vi "HEWH Check Voltage.vi"(8 "error in (no error)":errorcluster, 11 "UEF Calculated Values Input":T1 {"Data Indexes"."15 sec after Draw Index" format="%#.2f"; "Data Indexes"."15 sec after Draw Timestamp" format="%#.2f"; "Data Indexes"."Test Start Timestamp" format="%.2f"; "Data Indexes"."Test End Timestamp" format="%.2f"; "Data Indexes"."T0 Timestamp" format="%.2f"; "Data Indexes"."Tsf Timestamp" format="%.2f"; "Data Indexes"."Tsu0 Timestamp" format="%.2f"; "Data Indexes"."Tmax1 Timestamp" format="%.2f"; "Data Indexes"."Draw Index Timestamp" format="%#.2f"; "Data Indexes"."Non-Draw Timestamp" format="%#.2f"; "Data Indexes"."Heating Timestamp" format="%#.2f"; "Data Indexes"."Start Energy (BTU-Gas)" format="%.6f"; "Data Indexes"."Start Watt Hours" format="%.6f"; "Static Data"."V - Volume of Wh (True)" format="%.5f"; "Static Data"."T-Ambinet Nominal (°F)" format="%.5f"; "Static Data"."T-Inlet Setpoint (°F)" format="%.5f"; "Static Data"."T-Wh Setpoint (°F)" format="%.5f"; "Sampled Data"."Qe (Wh)" format="%.5f"; "Sampled Data"."Tau stby2 (hr)" format="%.5f"; "Sampled Data"."Tastby2 (°F)" format="%.5f"; "Sampled Data"."Qf (BTU)" format="%.5f"; "Sampled Data"."Qe (BTU)" format="%.5f"; "Sampled Data"."Tmax1 (°F)" format="%.5f"; "Sampled Data"."T0 (°F)" format="%.5f"; "Sampled Data"."Qr (BTU)" format="%.5f"; "Sampled Data"."T 24(°F)" format="%.5f"; "Sampled Data"."T astby(°F)" format="%.5f"; "Sampled Data"."T tstby(°F)" format="%.5f"; "Sampled Data"."T su0(°F)" format="%.5f"; "Sampled Data"."T suf(°F)" format="%.5f"; "Sampled Data"."Tau stby_1 (hr)" format="%.5f"; "Sampled Data"."Qsuf (BTU)" format="%.5f"; "Sampled Data"."Qsu0 (BTU)" format="%.5f"; "Calculated Values"."Draw Bonus Volume (gal)" format="%.6f"; "Calculated Values"."Adjustment Factor" format="%.6f"; "Calculated Values"."T*avg_del(n-1)" format="%.6f"; "Calculated Values"."T*min(n-1)" format="%.6f"; "Calculated Values"."T*avg_del(n)" format="%.6f"; "Calculated Values"."Vn" format="%.6f"; "Calculated Values"."Qdm (BTU)" format="%.6f"; "Calculated Values"."QHWD (BTU)" format="%.6f"; "Calculated Values"."QHW (BTU)" format="%.6f"; "Calculated Values"."UEF" format="%.6f"; "Calculated Values"."QHW67 (BTU)" format="%.6f"; "Calculated Values"."Qda (BTU)" format="%.6f"; "Calculated Values"."Qd (BTU)" format="%.6f"; "Calculated Values"."Q (BTU)" format="%.6f"; "Calculated Values"."UA (BTU/(hr*F))" format="%.6f"; "Calculated Values"."Qhr (BTU/hr)" format="%.6f"; "Calculated Values"."Qstby (BTU)" format="%.6f"; "Calculated Values"."nu_r" format="%.6f"; "Calculated Values"."CpUEF (BTU/(lb*F))" format="%.6f"; "Calculated Values"."rho_nu (lb/gal)" format="%.6f"; "Calculated Values"."V1- Vol (Gal)" format="%.6f"; "Calculated Values"."M cluster mass removed (lb)" format="%.6f"; "Calculated Values"."Cp theoretical (BTU/(lbm °F))" format="%.6f"; "Calculated Values"."Tin1 - Mean Inlet 1st Cluster (°F)" format="%.6f"; "Calculated Values"."Tdel1-Mean Outlet 1st Cluster(°F)" format="%.6f"; "Calculated Values"."Cp 24 (BTU/(lb*F))" format="%.6f"; "Calculated Values"."Cp standby (BTU/(lb*F))" format="%.6f"; "Calculated Values"."Cp2 (BTU/(lb*F))" format="%.6f"; "Calculated Values"."Cp1 (BTU/(lb*F))" format="%.6f"; "Calculated Values"."rho 24 (lb/gal)" format="%.6f"; "Calculated Values"."rho standby (lb/gal)" format="%.6f"; "Calculated Values"."rho 2 (lb/gal)" format="%.6f"; "Calculated Values"."Density of cold water All (lbm/gal)" format="%#.3g"; "Calculated Values"."CpHW (BTU/(lbm °F))" format="%#.3g"; "Calculated Values"."Density of hot water All (lbm/gal)" format="%#.3g"; "Calculated Values"."Mass of water All (lbm)" format="%#.3f"}) -> (0 "error out":errorcluster, 3 "UEF Calculated Values Output":T1 {"Data Indexes"."15 sec after Draw Index" format="%#.2f"; "Data Indexes"."15 sec after Draw Timestamp" format="%#.2f"; "Data Indexes"."Test Start Timestamp" format="%.2f"; "Data Indexes"."Test End Timestamp" format="%.2f"; "Data Indexes"."T0 Timestamp" format="%.2f"; "Data Indexes"."Tsf Timestamp" format="%.2f"; "Data Indexes"."Tsu0 Timestamp" format="%.2f"; "Data Indexes"."Tmax1 Timestamp" format="%.2f"; "Data Indexes"."Draw Index Timestamp" format="%#.2f"; "Data Indexes"."Non-Draw Timestamp" format="%#.2f"; "Data Indexes"."Heating Timestamp" format="%#.2f"; "Data Indexes"."Start Energy (BTU-Gas)" format="%.6f"; "Data Indexes"."Start Watt Hours" format="%.6f"; "Static Data"."V - Volume of Wh (True)" format="%.5f"; "Static Data"."T-Ambinet Nominal (°F)" format="%.5f"; "Static Data"."T-Inlet Setpoint (°F)" format="%.5f"; "Static Data"."T-Wh Setpoint (°F)" format="%.5f"; "Sampled Data"."Qe (Wh)" format="%.5f"; "Sampled Data"."Tau stby2 (hr)" format="%.5f"; "Sampled Data"."Tastby2 (°F)" format="%.5f"; "Sampled Data"."Qf (BTU)" format="%.5f"; "Sampled Data"."Qe (BTU)" format="%.5f"; "Sampled Data"."Tmax1 (°F)" format="%.5f"; "Sampled Data"."T0 (°F)" format="%.5f"; "Sampled Data"."Qr (BTU)" format="%.5f"; "Sampled Data"."T 24(°F)" format="%.5f"; "Sampled Data"."T astby(°F)" format="%.5f"; "Sampled Data"."T tstby(°F)" format="%.5f"; "Sampled Data"."T su0(°F)" format="%.5f"; "Sampled Data"."T suf(°F)" format="%.5f"; "Sampled Data"."Tau stby_1 (hr)" format="%.5f"; "Sampled Data"."Qsuf (BTU)" format="%.5f"; "Sampled Data"."Qsu0 (BTU)" format="%.5f"; "Calculated Values"."Draw Bonus Volume (gal)" format="%.6f"; "Calculated Values"."Adjustment Factor" format="%.6f"; "Calculated Values"."T*avg_del(n-1)" format="%.6f"; "Calculated Values"."T*min(n-1)" format="%.6f"; "Calculated Values"."T*avg_del(n)" format="%.6f"; "Calculated Values"."Vn" format="%.6f"; "Calculated Values"."Qdm (BTU)" format="%.6f"; "Calculated Values"."QHWD (BTU)" format="%.6f"; "Calculated Values"."QHW (BTU)" format="%.6f"; "Calculated Values"."UEF" format="%.6f"; "Calculated Values"."QHW67 (BTU)" format="%.6f"; "Calculated Values"."Qda (BTU)" format="%.6f"; "Calculated Values"."Qd (BTU)" format="%.6f"; "Calculated Values"."Q (BTU)" format="%.6f"; "Calculated Values"."UA (BTU/(hr*F))" format="%.6f"; "Calculated Values"."Qhr (BTU/hr)" format="%.6f"; "Calculated Values"."Qstby (BTU)" format="%.6f"; "Calculated Values"."nu_r" format="%.6f"; "Calculated Values"."CpUEF (BTU/(lb*F))" format="%.6f"; "Calculated Values"."rho_nu (lb/gal)" format="%.6f"; "Calculated Values"."V1- Vol (Gal)" format="%.6f"; "Calculated Values"."M cluster mass removed (lb)" format="%.6f"; "Calculated Values"."Cp theoretical (BTU/(lbm °F))" format="%.6f"; "Calculated Values"."Tin1 - Mean Inlet 1st Cluster (°F)" format="%.6f"; "Calculated Values"."Tdel1-Mean Outlet 1st Cluster(°F)" format="%.6f"; "Calculated Values"."Cp 24 (BTU/(lb*F))" format="%.6f"; "Calculated Values"."Cp standby (BTU/(lb*F))" format="%.6f"; "Calculated Values"."Cp2 (BTU/(lb*F))" format="%.6f"; "Calculated Values"."Cp1 (BTU/(lb*F))" format="%.6f"; "Calculated Values"."rho 24 (lb/gal)" format="%.6f"; "Calculated Values"."rho standby (lb/gal)" format="%.6f"; "Calculated Values"."rho 2 (lb/gal)" format="%.6f"; "Calculated Values"."Density of cold water All (lbm/gal)" format="%#.3g"; "Calculated Values"."CpHW (BTU/(lbm °F))" format="%#.3g"; "Calculated Values"."Density of hot water All (lbm/gal)" format="%#.3g"; "Calculated Values"."Mass of water All (lbm)" format="%#.3f"})   [LabVIEW 2023]
uses:
  Type Definitions/UEF Constants.ctl
  Type Definitions/HEWH Draw Stats.ctl
  Type Definitions/HEWH FHR Draw Type.ctl
  Type Definitions/FHR Bins.ctl
  Type Definitions/HEWH Meter Type.ctl
  Type Definitions/HEWH Seconds to Remove.ctl
  Type Definitions/HEWH Remove From Location.ctl
panel:
  # "FHR"
  # "FHR"
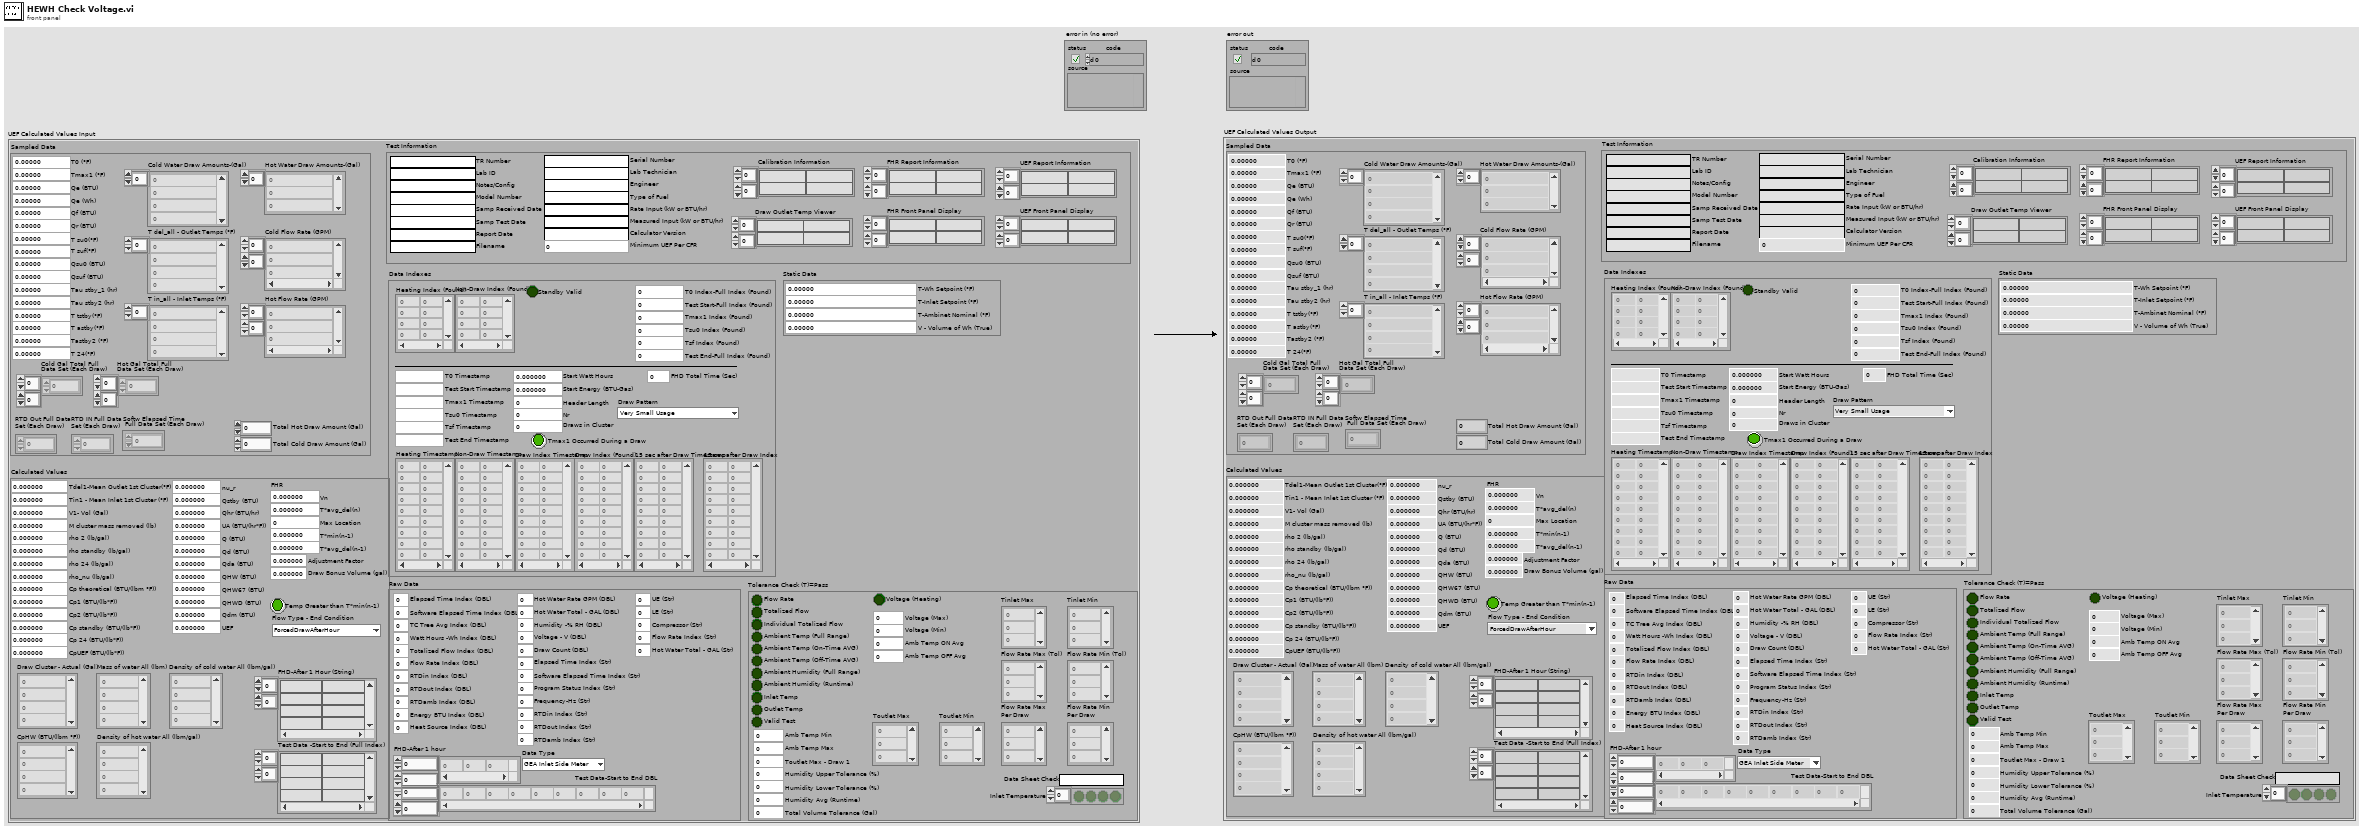
[diagram p1: front panel]
types:
  T1 = typedef "UEF Constants.ctl" = cluster{"Calculated Values":T2, "Sampled Data":cluster{"Cold Water Draw Amounts-(Gal)":dbl[], "T del_all - Outlet Temps (°F)":dbl[], "T in_all - Inlet Temps (°F)":dbl[], "Qsu0 (BTU)":dbl, "Qsuf (BTU)":dbl, "Tau stby_1 (hr)":dbl, "T suf(°F)":dbl, "T su0(°F)":dbl, "T tstby(°F)":dbl, "T astby(°F)":dbl, "T 24(°F)":dbl, "Qr (BTU)":dbl, "T0 (°F)":dbl, "Tmax1 (°F)":dbl, "Qe (BTU)":dbl, "Qf (BTU)":dbl, "Tastby2 (°F)":dbl, "RTD Out Full Data\nSet (Each Draw)":dbl[][], "RTD IN Full Data\nSet (Each Draw)":dbl[][], "Tau stby2 (hr)":dbl, "Hot Water Draw Amounts-(Gal)":dbl[], "Cold Flow Rate (GPM)":dbl[][], "Hot Flow Rate (GPM)":dbl[][], "Softw Elapsed Time\n Full Data Set (Each Draw)":dbl[][], "Cold Gal Total Full\nData Set (Each Draw)":dbl[][], "Total Hot Draw Amount (Gal) ":dbl, "Total Cold Draw Amount (Gal)":dbl, "Qe (Wh)":dbl, "Hot Gal Total Full\nData Set (Each Draw)":dbl[][]}, "Static Data":cluster{"T-Wh Setpoint (°F)":dbl, "T-Inlet Setpoint (°F)":dbl, "T-Ambinet Nominal (°F)":dbl, "V - Volume of Wh (True)":dbl}, "Data Indexes":cluster{"Test Start-Full Index (Found)":i32, "Header Length":i32, "Draw Index (Found)":i32[][], "Nr":i32, "Start Watt Hours":dbl, "Tsu0 Index (Found)":i32, "Tsf Index (Found)":i32, "Start Energy (BTU-Gas)":dbl, "Draws in Cluster":i32, "T0 Index-Full Index (Found)":i32, "Non-Draw Index (Found)":i32[][], "Tmax1 Index (Found)":i32, "Test End-Full Index (Found)":i32, "Heating Index (Found)":i32[][], "Heating Timestamp":dbl[][], "Non-Draw Timestamp":dbl[][], "Draw Index Timestamp":dbl[][], "Tmax1 Timestamp":dbl, "Tsu0 Timestamp":dbl, "Tsf Timestamp":dbl, "T0 Timestamp":dbl, "Test End Timestamp":dbl, "Test Start Timestamp":dbl, "15 sec after Draw Timestamp":dbl[][], "15 sec after Draw Index":dbl[][], "Tmax1 Occurred During a Draw":bool, "FHD Total Time (Sec)":dbl, "Draw Pattern":T4, "Standby Valid":bool}, "Raw Data":cluster{"Elapsed Time Index (DBL)":i32, "Software Elapsed Time Index (DBL)":i32, "TC Tree Avg Index (DBL)":i32, "Watt Hours -Wh Index (DBL)":i32, "Energy BTU Index (DBL)":i32, "Totalized Flow Index (DBL)":i32, "Flow Rate Index (DBL)":i32, "Program Status Index (Str)":i32, "RTDin Index (DBL)":i32, "RTDout Index (DBL)":i32, "RTDamb Index (DBL)":i32, "Test Data-Start to End DBL":dbl[][], "Data Type":T5, "Heat Source Index (DBL)":i32, "Hot Water Rate GPM (DBL)":i32, "Hot Water Total - GAL (DBL)":i32, "FHD-After 1 hour":dbl[][], "Humidity -% RH (DBL)":i32, "Voltage - V (DBL)":i32, "Draw Count (DBL)":i32, "Elapsed Time Index (Str)":i32, "Software Elapsed Time Index (Str)":i32, "Frequency-Hz (Str)":i32, "RTDin Index (Str)":i32, "RTDout Index (Str)":i32, "RTDamb Index (Str)":i32, "UE (Str)":i32, "LE (Str)":i32, "Compressor (Str)":i32, "Flow Rate Index (Str)":i32, "Hot Water Total - GAL (Str)":i32}, "Tolerance Check (T)=Pass":cluster{"Flow Rate":bool, "Totalized Flow":bool, "Ambient Temp (Full Range)":bool, "Ambient Humidity (Full Range)":bool, "Inlet Temp":bool, "Outlet Temp":bool, "Valid Test":bool, "Individual Totalized Flow":bool, "Data Sheet Check":string, "Inlet Temperature":bool[], "Tinlet Max":dbl[], "Tinlet Min":dbl[], "Flow Rate Max (Tol)":dbl[], "Flow Rate Min (Tol)":dbl[], "Amb Temp Max":dbl, "Amb Temp Min":dbl, "Toutlet Max - Draw 1":dbl, "Humidity Upper Tolerance (%)":dbl, "Total Volume Tolerance (Gal)":dbl, "Humidity Lower Tolerance (%)":dbl, "Flow Rate Max\nPer Draw":dbl[], "Flow Rate Min\nPer Draw":dbl[], "Ambient Humidity (Runtime)":bool, "Humidity Avg (Runtime)":dbl, "Ambient Temp (On-Time AVG)":bool, "Ambient Temp (Off-Time AVG)":bool, "Amb Temp OFF Avg":dbl, "Amb Temp ON Avg":dbl, "Voltage (Heating)":bool, "Voltage (Min)":dbl, "Voltage (Max)":dbl, "Toutlet Max":dbl[], "Toutlet Min":dbl[]}, "Test Information":cluster{"TR Number":string, "Lab ID":string, "Notes/Config":string, "Model Number":string, "Serial Number":string, "Lab Technician":string, "Engineer":string, "Type of Fuel":string, "Samp Received Date":string, "Samp Test Date":string, "Report Date":string, "Rate Input (kW or BTU/hr)":string, "Measured Input (kW or BTU/hr)":string, "Filename":string, "Calibration Information":string[][], "Calculator Version":string, "Minimum UEF Per CFR":dbl, "UEF Report Information":string[][], "FHR Report Information":string[][], "FHR Front Panel Display":string[][], "UEF Front Panel Display":string[][], "Draw Outlet Temp Viewer":string[][]}}
  T2 = typedef "HEWH Draw Stats.ctl" = cluster{"Draw Cluster - Actual (Gal)":dbl[], "Mass of water All (lbm)":dbl[], "Density of hot water All (lbm/gal)":dbl[], "CpHW (BTU/(lbm °F))":dbl[], "rho 2 (lb/gal)":dbl, "rho standby (lb/gal)":dbl, "rho 24 (lb/gal)":dbl, "Cp1 (BTU/(lb*F))":dbl, "Cp2 (BTU/(lb*F))":dbl, "Cp standby (BTU/(lb*F))":dbl, "Cp 24 (BTU/(lb*F))":dbl, "nu_r":dbl, "Qstby (BTU)":dbl, "Qhr (BTU/hr)":dbl, "UA (BTU/(hr*F))":dbl, "Q (BTU)":dbl, "Qd (BTU)":dbl, "Qda (BTU)":dbl, "QHW67 (BTU)":dbl, "UEF":dbl, "Tdel1-Mean Outlet 1st Cluster(°F)":dbl, "Tin1 - Mean Inlet 1st Cluster (°F)":dbl, "Cp theoretical (BTU/(lbm °F))":dbl, "M cluster mass removed (lb)":dbl, "V1- Vol (Gal)":dbl, "Test Data -Start to End (Full Index)":string[][], "rho_nu (lb/gal)":dbl, "Density of cold water All (lbm/gal)":dbl[], "CpUEF (BTU/(lb*F))":dbl, "QHW (BTU)":dbl, "QHWD (BTU)":dbl, "Qdm (BTU)":dbl, "FHD-After 1 Hour (String)":string[][], "Vn":dbl, "T*avg_del(n)":dbl, "Max Location":i32, "T*min(n-1)":dbl, "T*avg_del(n-1)":dbl, "Temp Greater than T*min(n-1)":bool, "Adjustment Factor":dbl, "Draw Bonus Volume (gal)":dbl, "Flow Type - End Condition":T3}
  T3 = typedef "HEWH FHR Draw Type.ctl" = enum16{"ForcedDrawAfterHour", "HeatingCutoffBeforeHour"}
  T4 = typedef "FHR Bins.ctl" = enum16{"Very Small Usage", "Low Usage", "Medium Usage", "High Usage", "Undefined"}
  T5 = typedef "HEWH Meter Type.ctl" = enum16{"GEA Inlet Side Meter", "GEA Outlet Side Meter", "CSA Inlet Side Meter"}
  T6 = typedef "HEWH Remove From Location.ctl" = enum16{"Remove from  Beginning", "Remove from End"}
  T7 = typedef "HEWH Seconds to Remove.ctl" = enum16{"5 Seconds", "15 Seconds"}
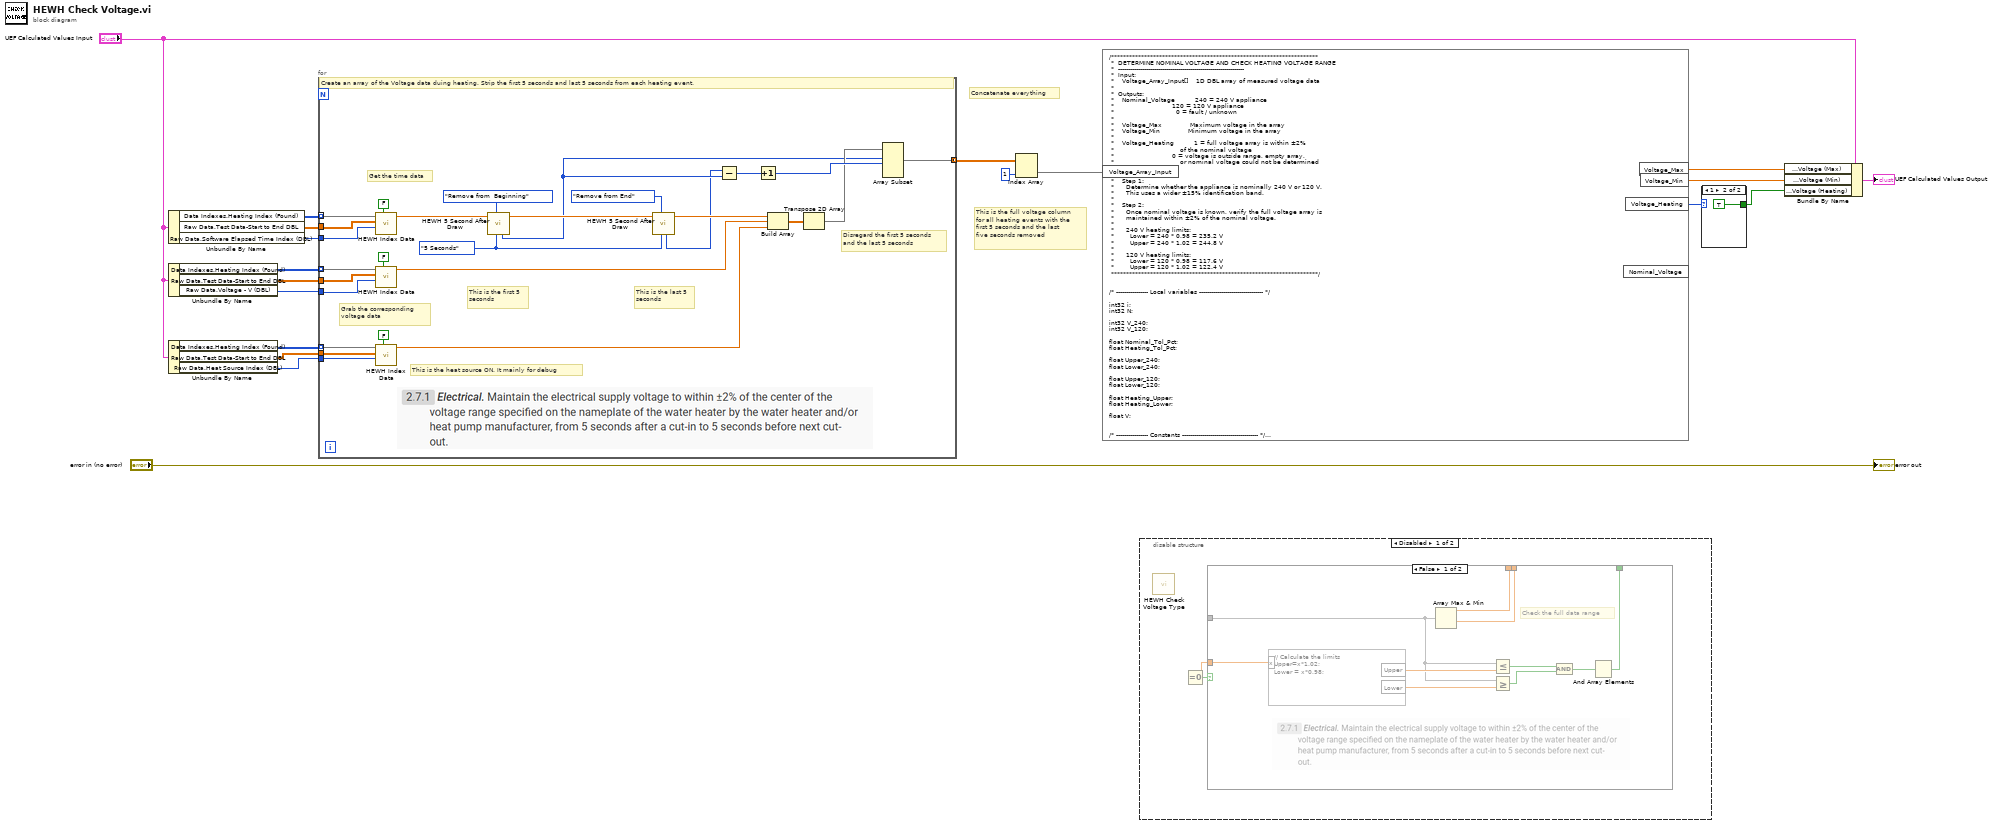
[diagram p0: block diagram]
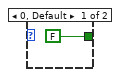
[diagram p2: hidden frame]
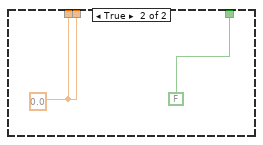
[diagram p3: hidden frame]
diagram:
  # "This is the full voltage column\nfor all heating events with the\nfirst 5 seconds and the last\nfive seconds removed"
  # "Concatenate everything"
  n1 = Unbundle By Name("UEF Calculated Values Input") -> ("Data Indexes.Heating Index (Found)"=w16:i32[][], "Raw Data.Test Data-Start to End DBL"=w15:dbl[][], "Raw Data.Software Elapsed Time Index (DBL)"=w14:i32)
  n2 = Unbundle By Name("UEF Calculated Values Input") -> ("Data Indexes.Heating Index (Found)"=w18:i32[][], "Raw Data.Test Data-Start to End DBL"=w19:dbl[][], "Raw Data.Voltage - V (DBL)"=w17:i32)
  n3 = Unbundle By Name("UEF Calculated Values Input") -> ("Data Indexes.Heating Index (Found)"=w13:i32[][], "Raw Data.Test Data-Start to End DBL"=w12:dbl[][], "Raw Data.Heat Source Index (DBL)"=w11:i32)
  n4 = for {
    tunnel: w19 -> [w45]
    tunnel: w18 -> [w44] mode=indexing
    tunnel: w17 -> [w43]
    tunnel: w16 -> [w41] mode=indexing
    tunnel: w15 -> [w40]
    tunnel: w14 -> [w39]
    tunnel: w13 -> [w35] mode=indexing
    tunnel: w12 -> [w34]
    tunnel: w11 -> [w33]
    tunnel: [w25] -> w10 mode=concatenating
    w22 = HEWH_Seconds_to_Remove."5 Seconds" ("Seconds to Remove")
    # "This is the heat source ON. It mainly for debug"
    # "This is the last 5\nseconds"
    # "This is the first 5\nseconds"
    # "Disregard the first 5 seconds\nand the last 5 seconds"
    # "Grab the corresponding \nvoltage data"
    # "Get the time data"
    # "Create an array of the Voltage data duing heating. Strip the first 5 seconds and last 5 seconds from each heating event."
    n5 = call "HEWH Index Data.vi"("Basic Index?"=FALSE, "Data Index Location"=w39, "Test Data-Start to End DBL"=w40, "Draw Index"=w41) -> ("Extracted Data"=w31:dbl[])  [unwired: 5 in, 2 out]
    n6 = call "HEWH Index Data.vi"("Basic Index?"=FALSE, "Data Index Location"=w43, "Test Data-Start to End DBL"=w45, "Draw Index"=w44) -> ("Extracted Data"=w38:dbl[])  [unwired: 5 in, 2 out]
    n7 = call "HEWH Index Data.vi"("Basic Index?"=FALSE, "Data Index Location"=w33, "Test Data-Start to End DBL"=w34, "Draw Index"=w35) -> ("Extracted Data"=w32:dbl[])  [unwired: 5 in, 2 out]
    n8 = call "HEWH 5 Second After Draw.vi"("Seconds to Remove"=w22, "Remove from location"=HEWH_Remove_From_Location."Remove from  Beginning", "Software Elapsed Time (s) in"=w31) -> ("Software Elapsed Time (s) out"=w30:dbl[], "Time Index"=w24:i32)  [unwired: 6 in, 1 out]
    n9 = call "HEWH 5 Second After Draw.vi"("Seconds to Remove"=w22, "Remove from location"=HEWH_Remove_From_Location."Remove from End", "Software Elapsed Time (s) in"=w30) -> ("Software Elapsed Time (s) out"=w29:dbl[], "Time Index"=w23:i32)  [unwired: 6 in, 1 out]
    n10 = Subtract(x=w23, y=w24) -> (x-y=w28:i32)
    n11 = Increment(x=w28) -> (x+1=w27:i32)
    n12 = Build Array(w29, w38, w32) -> (w37:dbl[][])
    n13 = Transpose 2D Array(2D array=w37) -> (transposed array=w26:dbl[][])
    n14 = Array Subset "Array Subset"(array=w26, index (row)=w24, length (row)=w27) -> (w25:dbl[][])  [unwired: 2 in]
  }
  n15 = Index Array(array=w10, index (col)=1 ("disabled index (col)")) -> (element=w6:dbl[])  [unwired: 1 in]
  n16 = formula code="/*********************************************************************\n *  DETERMINE NOMINAL VOLTAGE AND CHECK HEATING VOLTAGE RANGE\n *  ---------------------------------------------------------------\n *  Input:\n *    Voltage_Array_Input[]    1D DBL array of measured voltage data\n *\n *  Outputs:\n *    Nominal_Voltage          240 = 240 V appliance\n *                             120 = 120 V appliance\n *                               0 = fault / unknown\n *\n *    Voltage_Max              Maximum voltage in the array\n *    Voltage_Min              Minimum voltage in the array\n *\n *    Voltage_Heating          1 = full voltage array is within ±2%\n *                                 of the nominal voltage\n *                             0 = voltage is outside range, empty array,\n *                                 or nominal voltage could not be determined\n *\n *  Logic:\n *    Step 1:\n *      Determine whether the appliance is nominally 240 V or 120 V.\n *      This uses a wider ±15% identification band.\n *\n *    Step 2:\n *      Once nominal voltage is known, verify the full voltage array is\n *      maintained within ±2% of the nominal voltage.\n *\n *      240 V heating limits:\n *        Lower = 240 * 0.98 = 235.2 V\n *        Upper = 240 * 1.02 = 244.8 V\n *\n *      120 V heating limits:\n *        Lower = 120 * 0.98 = 117.6 V\n *        Upper = 120 * 1.02 = 122.4 V\n *********************************************************************/\n\n\n/* ---------------- Local variables -------------------------------- */\n\nint32 i;\nint32 N;\n\nint32 V_240;\nint32 V_120;\n\nfloat Nominal_Tol_Pct;\nfloat Heating_Tol_Pct;\n\nfloat Upper_240;\nfloat Lower_240;\n\nfloat Upper_120;\nfloat Lower_120;\n\nfloat Heating_Upper;\nfloat Heating_Lower;\n\nfloat V;\n\n\n/* ---------------- Constants -------------------------------------- */\n\nNominal_Tol_Pct = 0.15;     /* ±15% band used to identify voltage type */\nHeating_Tol_Pct = 0.02;     /* ±2% band used during heating check      */\n\n\n/* ---------------- Default outputs -------------------------------- */\n\nint32 Nominal_Voltage = 0.0;\n\nVoltage_Max = 0.0;\nVoltage_Min = 0.0;\n\nint32 Voltage_Heating = 0;  /* 0 = out of tolerance, 1 = within tolerance */\n\n\n/* ---------------- Get array length ------------------------------- */\n\nN = sizeOfDim(Voltage_Array_Input, 0);\n\n\n/* ---------------- Calculate nominal identification limits --------- */\n\nUpper_240 = 240.0 * (1.0 + Nominal_Tol_Pct);\nLower_240 = 240.0 * (1.0 - Nominal_Tol_Pct);\n\nUpper_120 = 120.0 * (1.0 + Nominal_Tol_Pct);\nLower_120 = 120.0 * (1.0 - Nominal_Tol_Pct);\n\n\n/* ---------------- Evaluate voltage data --------------------------- */\n\nif (N > 0)\n{\n    /*\n     * Initialize min and max using the first sample.\n     */\n\n    Voltage_Max = Voltage_Array_Input[0];\n    Voltage_Min = Voltage_Array_Input[0];\n\n\n    /*\n     * Start both nominal-voltage checks as TRUE.\n     * If any sample is outside a nominal range,\n     * set that range check to FALSE.\n     */\n\n    V_240 = 1;\n    V_120 = 1;\n\n\n    for (i = 0; i < N; i++)\n    {\n        V = Voltage_Array_Input[i];\n\n\n        /* Track maximum voltage */\n        if (V > Voltage_Max)\n        {\n            Voltage_Max = V;\n        }\n\n\n        /* Track minimum voltage */\n        if (V < Voltage_Min)\n        {\n            Voltage_Min = V;\n        }\n\n\n        /* Check 240 V nominal range */\n        if (V < Lower_240 || V > Upper_240)\n        {\n            V_240 = 0;\n        }\n\n\n        /* Check 120 V nominal range */\n        if (V < Lower_120 || V > Upper_120)\n        {\n            V_120 = 0;\n        }\n    }\n\n\n    /*\n     * Select final nominal voltage.\n     *\n     * Valid:\n     *   V_240 = 1 and V_120 = 0  --> 240 V\n     *   V_240 = 0 and V_120 = 1  --> 120 V\n     *\n     * Fault:\n     *   V_240 = 1 and V_120 = 1\n     *   V_240 = 0 and V_120 = 0\n     */\n\n    if (V_240 == 1 && V_120 == 0)\n    {\n        Nominal_Voltage = 240.0;\n    }\n    else if (V_240 == 0 && V_120 == 1)\n    {\n        Nominal_Voltage = 120.0;\n    }\n    else\n    {\n        Nominal_Voltage = 0.0;\n    }\n\n\n    /*****************************************************************\n     * Heating voltage check.\n        Use Voltage_Min and Voltage_Max:\n     *\n     *   Voltage_Min >= Lower limit\n     *   Voltage_Max <= Upper limit\n     *\n     * If both are true, the full array is inside the allowed range.\n     *****************************************************************/\n\n    if (Nominal_Voltage > 0.0)\n    {\n        Heating_Upper = Nominal_Voltage * (1.0 + Heating_Tol_Pct);\n        Heating_Lower = Nominal_Voltage * (1.0 - Heating_Tol_Pct);\n\n        if (Voltage_Min >= Heating_Lower && Voltage_Max <= Heating_Upper)\n        {\n            Voltage_Heating = 1;\n        }\n        else\n        {\n            Voltage_Heating = 0;\n        }\n    }\n    else\n    {\n        /*\n         * Nominal voltage could not be determined.\n         * Treat heating voltage check as failed.\n         */\n\n        Voltage_Heating = 0;\n    }\n}\nelse\n{\n    /*\n     * Empty array fault.\n     */\n\n    Nominal_Voltage = 0.0;\n\n    Voltage_Max = 0.0;\n    Voltage_Min = 0.0;\n\n    Voltage_Heating = 0;\n}"("Voltage_Array_Input"=w6) -> ("Voltage_Max"=w4:dbl, "Voltage_Min"=w3:dbl, "Voltage_Heating"=w5:i32)  [unwired: 1 out]
  n17 = disable-structure shown="Disabled" {
    frame Disabled {
      n18 = call "HEWH Check Voltage Type.vi"() -> ()  [unwired: 8 in, 4 out]
      n19 = Equal To 0?() -> (x=w48:dbl, x = 0?=w49:bool)
      n20 = case shown="False" w49 {
        tunnel: w48 -> [w54 _]
        tunnel: [w52 _] -> w47
        tunnel: [w53 FALSE] -> _
        tunnel: [w51 w60] -> _
        tunnel: [w50 w60] -> _
        frame False {
          # "Check the full data range"
          n21 = formula code="// Calculate the limits\nUpper=x*1.02;\nLower = x*0.98;"("x"=w54) -> ("Upper"=w56:dbl, "Lower"=w55:dbl)
          n22 = Array Max & Min(array=w52) -> (max value=w51:dbl, min value=w50:dbl)  [unwired: 2 out]
          n23 = Less Or Equal?(x=w52, y=w56) -> (x <= y?=w57:bool)
          n24 = Greater Or Equal?(x=w52, y=w55) -> (x >= y?=w58:bool)
          n25 = And(x=w57, y=w58) -> (x .and. y?=w59:bool)
          n26 = And Array Elements(Boolean array=w59) -> (logical AND=w53:bool)
        }
        frame True {
          w60 = 0.0
        }
      }
    }
    frame Enabled {
    }
  }
  n27 = case shown="1" w5 {
    tunnel: [FALSE TRUE] -> w2
    frame 0, Default {
    }
    frame 1 {
    }
  }
  n28 = Bundle By Name(cluster="UEF Calculated Values Input", "Tolerance Check (T)=Pass.Voltage (Max)"=w4, "Tolerance Check (T)=Pass.Voltage (Min)"=w3, "Tolerance Check (T)=Pass.Voltage (Heating)"=w2) -> (→"UEF Calculated Values Output":T1)
  "error out" <- "error in (no error)"
